vi "MAXSONAR.vi"() -> ()   [LabVIEW 2021]
uses:
  <vilib>/myRIO/Instrument Drivers/Onboard IO/UART/typedef/VISA Configuration.ctl
  <vilib>/Platform/TimedLoop/XDataNode/timing_clust.ctl
  <vilib>/Platform/TimedLoop/XDataNode/nitl_modes.ctl
  <vilib>/Platform/TimedLoop/XDataNode/wakeup.ctl
  <vilib>/Instr/_visa.llb/VISA Configure Serial Port (Instr).vi
  <vilib>/platform/TimedLoop/XDataNode/XDataNode.xnode
  <vilib>/Platform/TimedLoop/XDataNode/XDNodeRunTimeDep.lvlib
  <vilib>/myRIO/Instrument Drivers/Onboard IO/UART/UART.lvlib
panel:
  out "error out":errorcluster
  in  "error in (no error)":errorcluster
  out "Characters Read":string
  in  "stop":bool
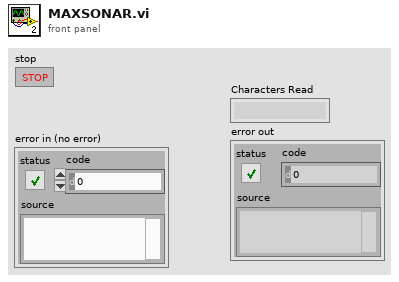
[diagram p1: front panel]
types:
  T1 = typedef "UART.lvlib/VISA Configuration.ctl" = cluster{"baud rate (9600)":u32, "data bits (8)":u16, "parity (0:none)":enum16{"None", "Odd", "Even", "Mark", "Space"}, "stop bits (10: 1 bit)":u16, "flow control (0:none)":u16, "termination char\n(0xA = '\\n' = LF) ":u8, "Enable Termination\nChar (T)":bool, "timeout (10sec)":u32}
  T2 = typedef "XDNodeRunTimeDep.lvlib/timing_clust.ctl" = cluster{"Expected End [f-1]":u64, "Actual End [f-1]":u64, "Finished Late? [f-1]":bool, "Expected End [i-1]":u64, "Actual End [i-1]":u64, "Finished Late? [i-1]":bool, "Expected Start [i]":u64, "Actual Start [i]":u64, "Expected Start [f]":u64, "Actual Start [f]":u64, "Source Name":string, "Structure Name":string, "Period":i64, "Deadline":i64, "Offset":i64, "Start":i64, "Priority":i32, "Timeout":i32, "Mode":T3, "Wakeup Reason":T4, "Error":errorcluster, "Source Type":string, "Secondary Source Type":string, "Global End Time":u64, "Global Start Time":u64, "Frame Duration":u64, "Iteration Duration":u64, "Assigned CPU":i32, "I/O Scan Engine Mode":u32}
  T3 = typedef "XDNodeRunTimeDep.lvlib/nitl_modes.ctl" = enum32{"No Change", "Process missed periods, maintain original phase", "Discard missed periods, maintain original phase", "Process missed periods, ignore original phase", "Discard missed periods, ignore original phase"}
  T4 = typedef "XDNodeRunTimeDep.lvlib/wakeup.ctl" = enum32{"Normal", "Aborted", "Asynchronous wakeup", "Timing source error", "Timed loop error", "Timeout"}
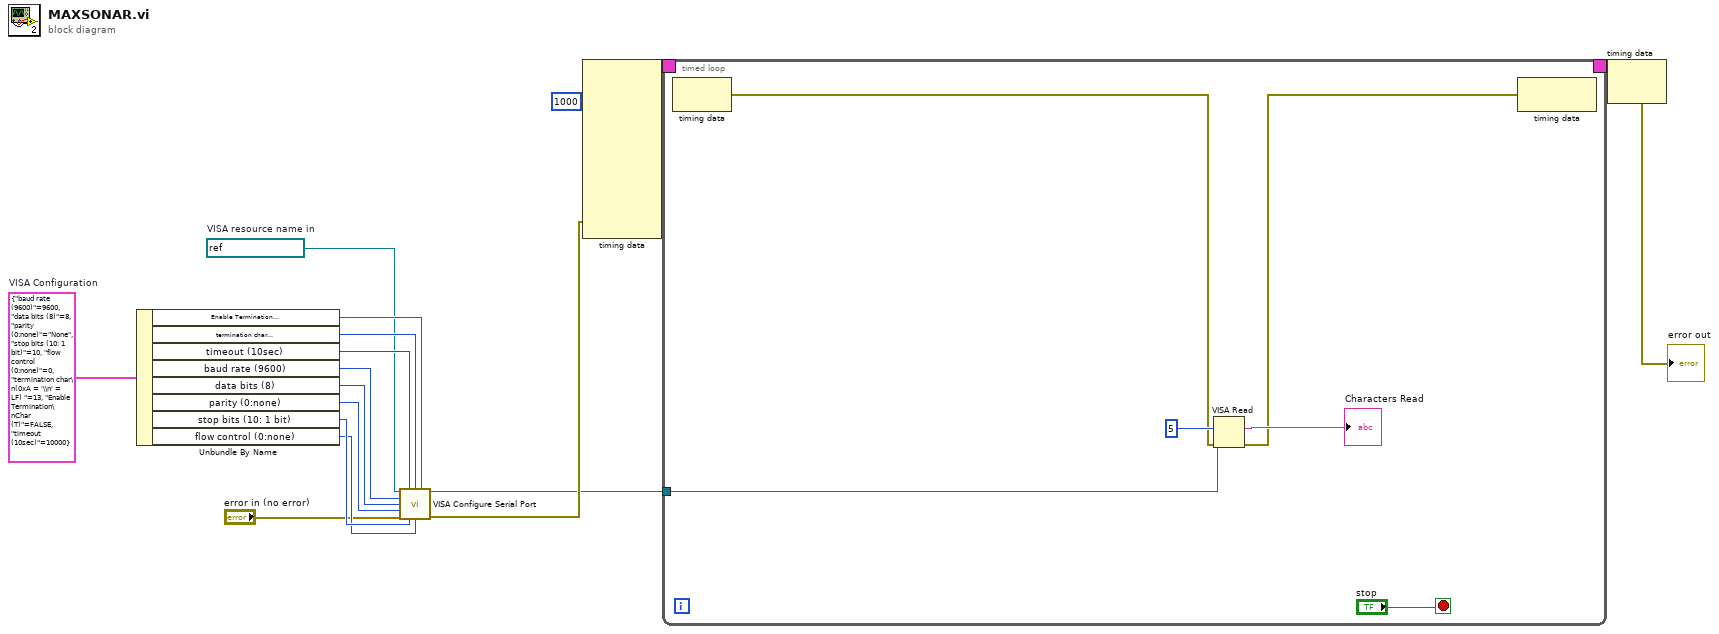
[diagram p0: block diagram]
diagram:
  w5 = T1 {"baud rate (9600)"=9600, "data bits (8)"=8, "parity (0:none)"=enum."None", "stop bits (10: 1 bit)"=10, "flow control (0:none)"=0, "termination char\n(0xA = '\\n' = LF) "=13, "Enable Termination\nChar (T)"=FALSE, "timeout (10sec)"=10000}  # VISA Configuration
  w4 = refnum<visa-resource-name> "ASRL2::INSTR"  # VISA resource name in
  n1 = Unbundle By Name(w5) -> ("Enable Termination\nChar (T)"=w6:bool, "termination char\n(0xA = '\\n' = LF)"=w7:u8, "timeout (10sec)"=w8:u32, "baud rate (9600)"=w13:u32, "data bits (8)"=w12:u16, "parity (0:none)"=w11:enum16{"None", "Odd", "Even", "Mark", "Space"}, "stop bits (10: 1 bit)"=w10:u16, "flow control (0:none)"=w9:u16)
  n2 = call-poly "VISA Configure Serial Port"("VISA resource name"=w4, "timeout (10sec)"=w8, "termination char\n(0xA = '\\n' = LF)"=w7, "Enable Termination\nChar (T)"=w6, "baud rate (9600)"=w13, "data bits (8)"=w12, "parity (0:none)"=w11, "error in (no error)"="error in (no error)", "stop bits (10: 1 bit)"=w10, "flow control (0:none)"=w9) -> ("VISA resource name out"=w1:refnum<visa-resource-name>, "error out"=w2:errorcluster)  [unwired: 4 in]
  n3 = node-c288(i64 1000 ("Period"), w2) -> (w17:T2)  [unwired: 8 in]
  n4 = timed-loop {
    timing: w17 -> [_]
    timing-out: [_] -> w16
    tunnel: w1 -> [w20]
    stop <- "stop" stop-if-true
    n5 = node-c288() -> (w18:errorcluster)  [unwired: 1 in]
    n6 = VISA Read(VISA resource name=w20, byte count=u32 5, error in (no error)=w18) -> (read buffer=→"Characters Read":string, error out=w21:errorcluster)  [unwired: 2 out]
    n7 = node-c288(w21) -> ()  [unwired: 1 out]
  }
  n8 = node-c288(w16) -> (→"error out":errorcluster)
